vi "StartAutoandGcode.vi"() -> ()   [LabVIEW 2014, in "LibraryGcode.lvlib"]
uses:
  LibraryGcode.lvlib
  ControlGlobal/stateModeDevice.ctl
  control/stateBoardFirmware.ctl
panel:
  out "LeapJog":cluster{"X":sgl, "Y":sgl, "Z":sgl}
  in  "DataGetFromSerial":string
  in  "stateBoardFirmware":T1=enum."Pos"
  in  "EMG":bool
  out "StateModeSoftWare":T2=enum."Config"
  out "G-Code Array 2":string[](array[string])=["Loi khong ket noChua Chon File"]
  in  "Start Auto":bool
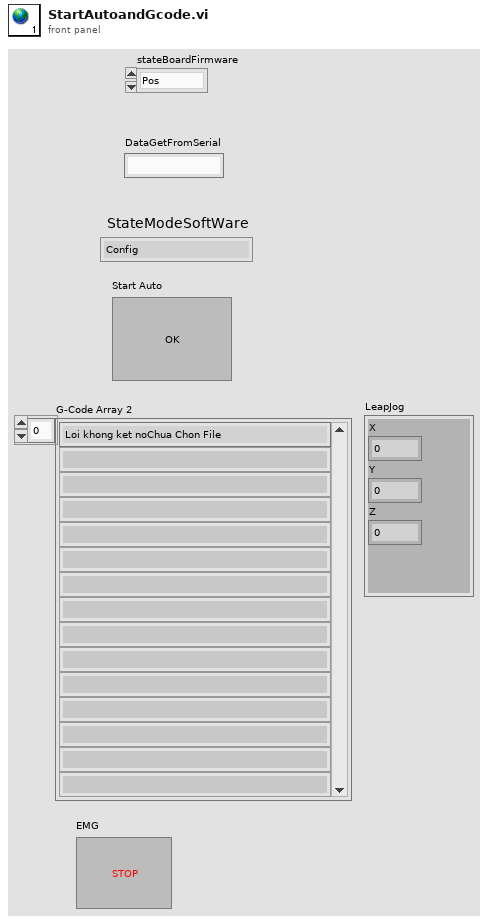
[diagram p1: front panel]
types:
  T1 = typedef "LibraryGcode.lvlib/stateBoardFirmware.ctl" = enum16{"Running", "Waiting", "Pos", "IDLE"}
  T2 = typedef "stateModeDevice.ctl" = enum16{"Auto", "Menu", "WaitAutoFinish", "Config", "initAuto"}
diagram:
